vi "Eat.vi"(8 "error in (no error)":errorcluster, 11 "Philosopher in":refnum<class "Philosopher.lvclass">) -> (0 "error out":errorcluster, 3 "Philosopher out":refnum<class "Philosopher.lvclass">)   [LabVIEW 2023, in "Philosopher.lvlib" / "Philosopher.lvclass"]
uses:
  Philosopher.lvclass
  Philosopher Statechart.lvsc/Trigger.ctl
  Philosopher.lvclass/Philosopher.ctl
  <vilib>/Statechart/Nodes/EventFiring/NI_SC_EventFiringNode.xnode
  Philosopher Statechart.lvsc
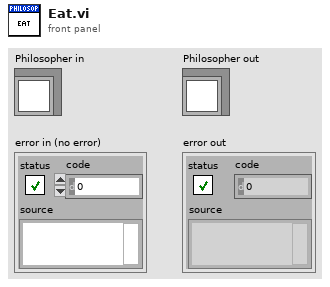
[diagram p1: front panel]
types:
  T1 = typedef "Philosopher.lvlib/Philosopher Statechart.lvsc/Trigger.ctl" = enum16{"NULL", "TIMEOUT", "EXIT", "EAT"}
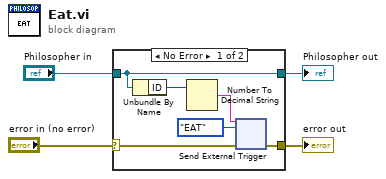
[diagram p0: block diagram]
diagram:
  n1 = case shown="No Error" "error in (no error)" {
    selector: "error in (no error)" -> [w6 w28]
    tunnel: [w5 w28] -> w3
    tunnel: [w10 w27] -> w1
    tunnel: "Philosopher in" -> [w10 w27]
    frame No Error {
      n2 = Unbundle By Name(w10) -> ("ID"=w9:i32)
      n3 = Number To Decimal String(number=w9) -> (decimal integer string=w8:string)  [unwired: 1 in]
      n4 = xnode "Send External Trigger"("Instance Name"=w8, "Trigger"=Trigger."EAT", "error in (no error)"=w6) -> ("error out"=w5:errorcluster)  [unwired: 1 out]
    }
    frame Error {
    }
  }
  "error out" <- w3
  "Philosopher out" <- w1
